vi "IO Channel Menu.vi"() -> ()   [LabVIEW 2013]
panel:
  in  "Enable Y Output":bool
  in  "Y Output":tag
  in  "Enable Y Input":bool
  in  "Y Input":tag
  in  "Enable X Output":bool
  in  "X Output":tag
  in  "Enable X Input":bool
  in  "X Input":tag
  in  "Division Input":tag
  in  "Sum Input":tag
  in  "Z Output":tag
  in  "Z Input":tag
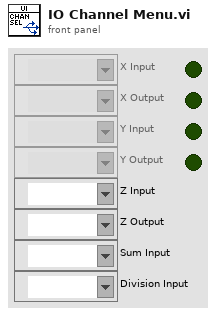
[diagram p1: front panel]
types:
  T1 = enum8{"Enabled", "Disabled", "Disabled and Grayed Out"}
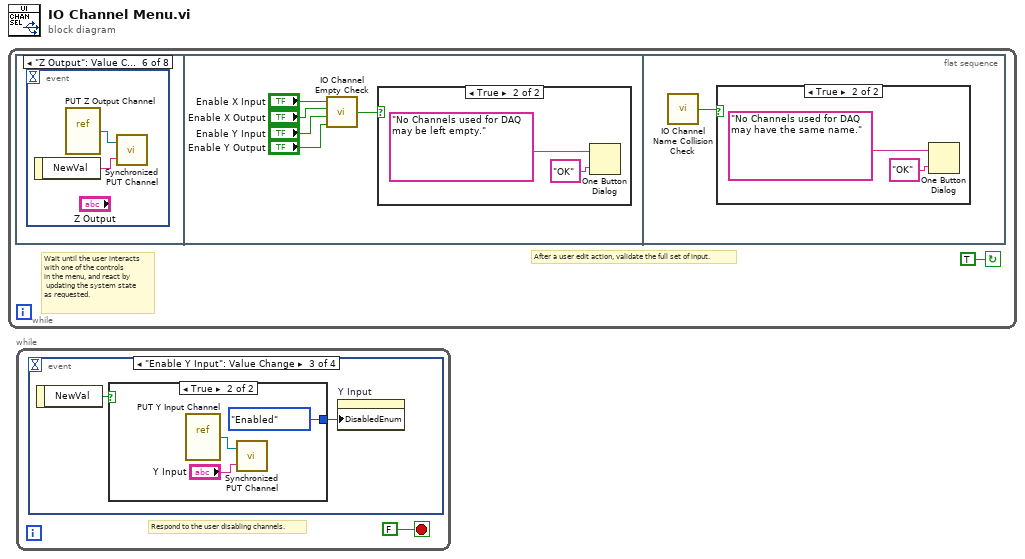
[diagram p0: block diagram]
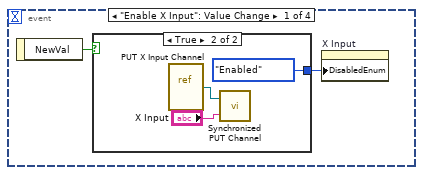
[diagram p2: hidden frame]
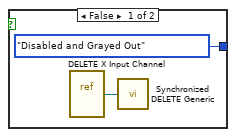
[diagram p3: hidden frame]
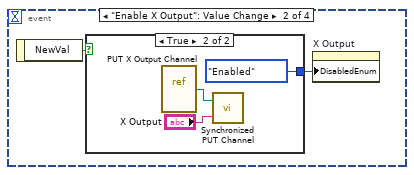
[diagram p4: hidden frame]
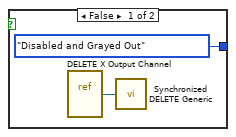
[diagram p5: hidden frame]
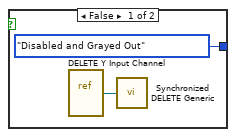
[diagram p6: hidden frame]
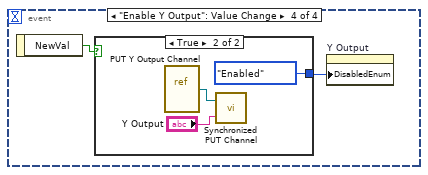
[diagram p7: hidden frame]
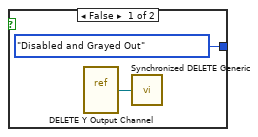
[diagram p8: hidden frame]
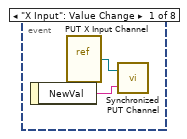
[diagram p9: hidden frame]
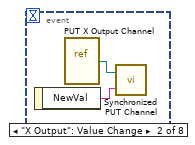
[diagram p10: hidden frame]
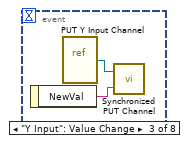
[diagram p11: hidden frame]
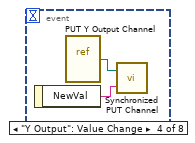
[diagram p12: hidden frame]
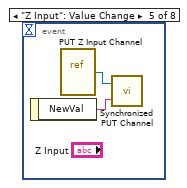
[diagram p13: hidden frame]
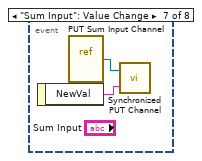
[diagram p14: hidden frame]
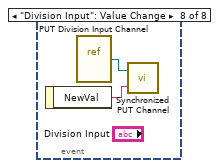
[diagram p15: hidden frame]
diagram:
  n1 = while {
    stop <- TRUE continue-if-true
    # "Wait until the user interacts \nwith one of the controls \nin the menu, and react by\n updating the system state \nas requested."
    # "After a user edit action, validate the full set of input."
    n2 = flat-sequence {
      frame #0 {
        n3 = event shown="[5] \"Z Output\": Value Change" {
          selector: _ -> [_ _ _ _ _ _ _ _]
          dyn-events: _ -> [_ _ _ _ _ _ _ _]
          timeout: _ -> [_ _ _ _ _ _ _ _]
          event "X Input": Value Change {
            n4 = event-data() -> ("NewVal"=w2:tag)  [unwired: 1 in]
            n5 = vi-ref "PUT X Input Channel.vi"() -> (w3:refnum<vi>)
            n6 = call "Synchronized PUT Channel.vi"("PUT Value"=w2, "PUT VI Reference"=w3) -> ()  [unwired: 1 in]
          }
          event "X Output": Value Change {
            n7 = event-data() -> ("NewVal"=w4:tag)  [unwired: 1 in]
            n8 = vi-ref "PUT X Output Channel.vi"() -> (w5:refnum<vi>)
            n9 = call "Synchronized PUT Channel.vi"("PUT Value"=w4, "PUT VI Reference"=w5) -> ()  [unwired: 1 in]
          }
          event "Y Input": Value Change {
            n10 = event-data() -> ("NewVal"=w6:tag)  [unwired: 1 in]
            n11 = vi-ref "PUT Y Input Channel.vi"() -> (w7:refnum<vi>)
            n12 = call "Synchronized PUT Channel.vi"("PUT Value"=w6, "PUT VI Reference"=w7) -> ()  [unwired: 1 in]
          }
          event "Y Output": Value Change {
            n13 = event-data() -> ("NewVal"=w8:tag)  [unwired: 1 in]
            n14 = vi-ref "PUT Y Output Channel.vi"() -> (w9:refnum<vi>)
            n15 = call "Synchronized PUT Channel.vi"("PUT Value"=w8, "PUT VI Reference"=w9) -> ()  [unwired: 1 in]
          }
          event "Z Input": Value Change {
            n16 = event-data() -> ("NewVal"=w10:tag)  [unwired: 1 in]
            n17 = vi-ref "PUT Z Input Channel.vi"() -> (w11:refnum<vi>)
            n18 = call "Synchronized PUT Channel.vi"("PUT Value"=w10, "PUT VI Reference"=w11) -> ()  [unwired: 1 in]
          }
          event "Z Output": Value Change {
            n19 = event-data() -> ("NewVal"=w12:tag)  [unwired: 1 in]
            n20 = vi-ref "PUT Z Output Channel.vi"() -> (w13:refnum<vi>)
            n21 = call "Synchronized PUT Channel.vi"("PUT Value"=w12, "PUT VI Reference"=w13) -> ()  [unwired: 1 in]
          }
          event "Sum Input": Value Change {
            n22 = event-data() -> ("NewVal"=w14:tag)  [unwired: 1 in]
            n23 = vi-ref "PUT Sum Input Channel.vi"() -> (w15:refnum<vi>)
            n24 = call "Synchronized PUT Channel.vi"("PUT Value"=w14, "PUT VI Reference"=w15) -> ()  [unwired: 1 in]
          }
          event "Division Input": Value Change {
            n25 = event-data() -> ("NewVal"=w16:tag)  [unwired: 1 in]
            n26 = vi-ref "PUT Division Input Channel.vi"() -> (w17:refnum<vi>)
            n27 = call "Synchronized PUT Channel.vi"("PUT Value"=w16, "PUT VI Reference"=w17) -> ()  [unwired: 1 in]
          }
        }
      }
      frame #1 {
        n28 = call "IO Channel Empty Check.vi"("Enable Y Output"="Enable Y Output", "Enable Y Input"="Enable Y Input", "Enable X Output"="Enable X Output", "Enable X Input"="Enable X Input") -> ("Required Channels Empty"=w22:bool)
        n29 = case shown="True" w22 {
          frame False {
          }
          frame True {
            n30 = One Button Dialog(message="No Channels used for DAQ may be left empty.", button name ("OK")="OK") -> ()  [unwired: 1 out]
          }
        }
      }
      frame #2 {
        n31 = call "IO Channel Name Collision Check.vi"() -> ("Channel Names Collide"=w25:bool)
        n32 = case shown="True" w25 {
          frame False {
          }
          frame True {
            n33 = One Button Dialog(message="No Channels used for DAQ may have the same name.", button name ("OK")="OK") -> ()  [unwired: 1 out]
          }
        }
      }
    }
  }
  n34 = while {
    stop <- FALSE stop-if-true
    # "Respond to the user disabling channels."
    n35 = event shown="[2] \"Enable Y Input\": Value Change" {
      selector: _ -> [_ _ _ _]
      dyn-events: _ -> [_ _ _ _]
      timeout: _ -> [_ _ _ _]
      event "Enable X Input": Value Change {
        n36 = event-data() -> ("NewVal"=w30:bool)  [unwired: 1 in]
        n37 = case shown="True" w30 {
          tunnel: [T1."Disabled and Grayed Out" ("Disabled") T1."Enabled" ("Disabled")] -> w29
          frame False {
            n38 = vi-ref "DELETE X Input Channel.vi"() -> (w31:refnum<vi>)
            n39 = call "Synchronized DELETE Generic.vi"("DEL VI Reference"=w31) -> ()
          }
          frame True {
            n40 = vi-ref "PUT X Input Channel.vi"() -> (w34:refnum<vi>)
            n41 = call "Synchronized PUT Channel.vi"("PUT Value"="X Input", "PUT VI Reference"=w34) -> ()  [unwired: 1 in]
          }
        }
        n42 = property on="X Input" class="DAQmxName"("DisabledEnum"=w29) -> ()  [unwired: 2 in, 2 out]
      }
      event "Enable X Output": Value Change {
        n43 = event-data() -> ("NewVal"=w36:bool)  [unwired: 1 in]
        n44 = case shown="True" w36 {
          tunnel: [T1."Disabled and Grayed Out" ("Disabled") T1."Enabled" ("Disabled")] -> w37
          frame False {
            n45 = vi-ref "DELETE X Output Channel.vi"() -> (w38:refnum<vi>)
            n46 = call "Synchronized DELETE Generic.vi"("DEL VI Reference"=w38) -> ()
          }
          frame True {
            n47 = vi-ref "PUT X Output Channel.vi"() -> (w41:refnum<vi>)
            n48 = call "Synchronized PUT Channel.vi"("PUT Value"="X Output", "PUT VI Reference"=w41) -> ()  [unwired: 1 in]
          }
        }
        n49 = property on="X Output" class="DAQmxName"("DisabledEnum"=w37) -> ()  [unwired: 2 in, 2 out]
      }
      event "Enable Y Input": Value Change {
        n50 = event-data() -> ("NewVal"=w43:bool)  [unwired: 1 in]
        n51 = case shown="True" w43 {
          tunnel: [T1."Disabled and Grayed Out" ("Disabled") T1."Enabled" ("Disabled")] -> w44
          frame False {
            n52 = vi-ref "DELETE Y Input Channel.vi"() -> (w45:refnum<vi>)
            n53 = call "Synchronized DELETE Generic.vi"("DEL VI Reference"=w45) -> ()
          }
          frame True {
            n54 = vi-ref "PUT Y Input Channel.vi"() -> (w48:refnum<vi>)
            n55 = call "Synchronized PUT Channel.vi"("PUT Value"="Y Input", "PUT VI Reference"=w48) -> ()  [unwired: 1 in]
          }
        }
        n56 = property on="Y Input" class="DAQmxName"("DisabledEnum"=w44) -> ()  [unwired: 2 in, 2 out]
      }
      event "Enable Y Output": Value Change {
        n57 = event-data() -> ("NewVal"=w50:bool)  [unwired: 1 in]
        n58 = case shown="True" w50 {
          tunnel: [T1."Disabled and Grayed Out" ("Disabled") T1."Enabled" ("Disabled")] -> w51
          frame False {
            n59 = vi-ref "DELETE Y Output Channel.vi"() -> (w52:refnum<vi>)
            n60 = call "Synchronized DELETE Generic.vi"("DEL VI Reference"=w52) -> ()
          }
          frame True {
            n61 = vi-ref "PUT Y Output Channel.vi"() -> (w55:refnum<vi>)
            n62 = call "Synchronized PUT Channel.vi"("PUT Value"="Y Output", "PUT VI Reference"=w55) -> ()  [unwired: 1 in]
          }
        }
        n63 = property on="Y Output" class="DAQmxName"("DisabledEnum"=w51) -> ()  [unwired: 2 in, 2 out]
      }
    }
  }
